vi "Remove Comments.vi"(8 "error in (no error)":errorcluster, 11 "input string":string="{\n\"Cluster\": {\n\"Name\": \"test\", //Represents the name of a person\n\"Department\": \"test2\",/*Gives the department name and \nthe functionality of the department*/\n\"NewElement\": \"test\"/*test*/\n}") -> (0 "error out":errorcluster, 2 "Number of comments":i32, 3 "output String":string)   [LabVIEW 2015]
doc: "This VI removes comments from the JSON that has just been read from a JSON file.This step is mandatory before parsing out the data to the next step. \nIt is capable of removing <b>single line ( // // ) </b>and<b> multiple line (/* */)</b>comments from the input JSON String."
panel:
  # "The input can be changed to test the working of the SubVI"
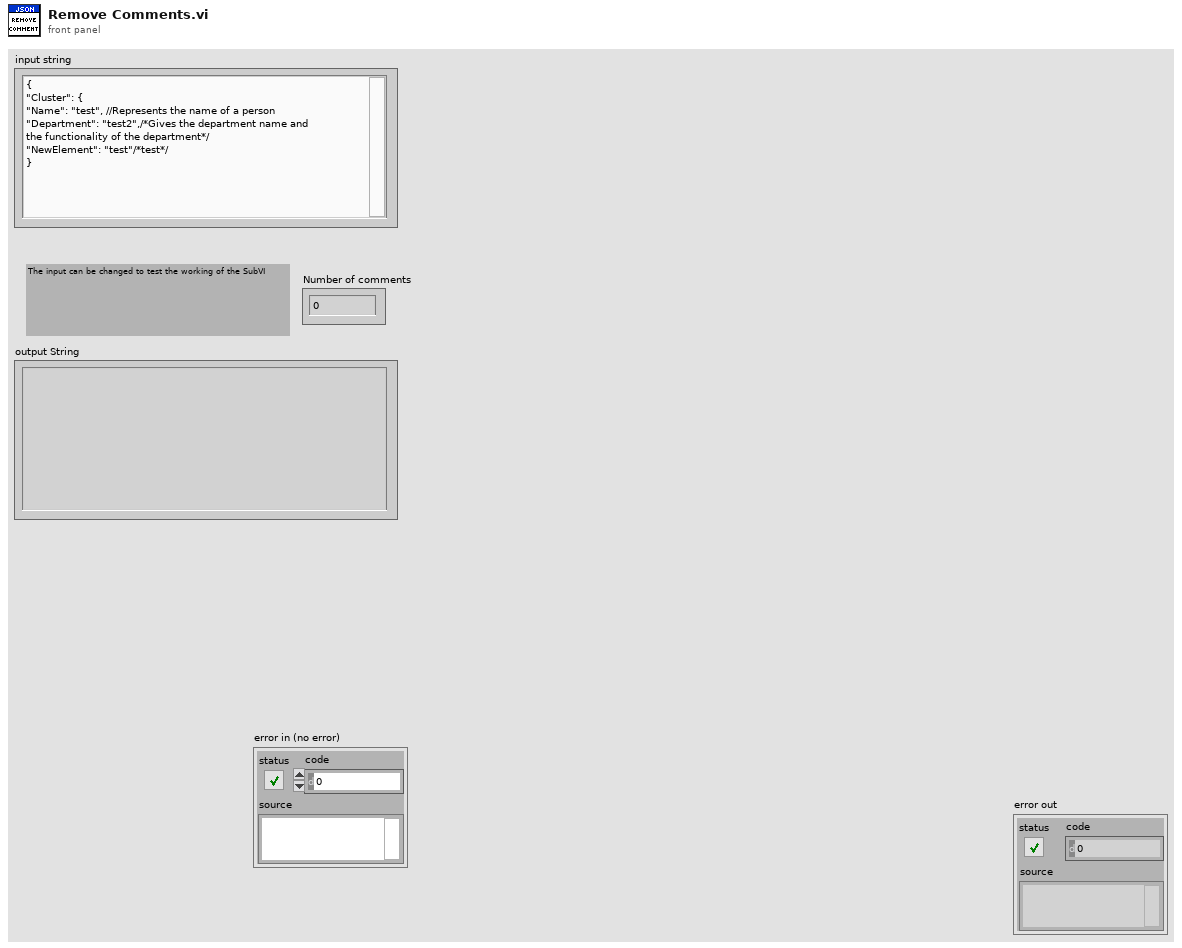
[diagram p1: front panel]
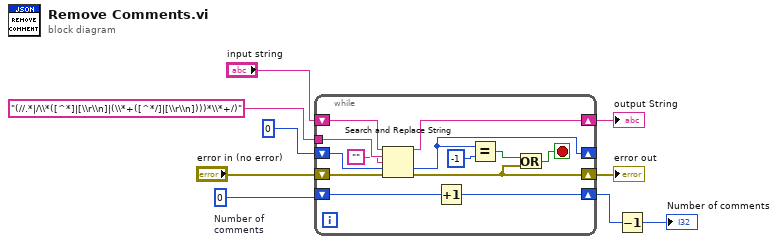
[diagram p0: block diagram]
diagram:
  w3 = u64 0  # Number of comments
  n1 = while {
    tunnel: "(//.*|/\\*([^*]|[\\r\\n]|(\\*+([^*/]|[\\r\\n])))*\\*+/)" ("regular expression") -> [w22]
    shift-right: [w11] -> w8
    shift-left: "error in (no error)" -> [w17]
    shift-right: [w15] -> _
    shift-left: 0 ("offset past match") -> [w19]
    shift-right: [w20] -> w6
    shift-left: "input string" -> [w18]
    shift-right: [w13] -> w4
    shift-left: w3 -> [w14]
    stop <- w10 stop-if-true
    n2 = Search and Replace String(input string=w18, search string=w22, replace string="", offset=w19, error in=w17) -> (result string=w20:string, offset past replacement=w15:i32, error out=w11:errorcluster)  [unwired: 3 in, 1 out]
    n3 = Increment(x=w14) -> (x+1=w13:u64)
    n4 = Equal?(x=w15, y=-1) -> (x = y?=w12:bool)
    n5 = Or(x=w12, y=w11) -> (x .or. y?=w10:bool)
  }
  "error out" <- w8
  "output String" <- w6
  n6 = Decrement(x=w4) -> (x-1=→"Number of comments":u64)
